vi "Read Line detector configuration.vi"(8 "error in (no error)":errorcluster, 11 "Line Detector in":refnum<class "Resonance Detector.lvclass">) -> (0 "error out":errorcluster, 2 "Configuration":T1={"Peak width guess"=0.0, "Background removal"=enum."NONE", "Smoothing"=enum."NONE", "Smooth window"=100.0, "Relative threshold"=0.0, "Finder algorithm"=enum."Basic", "Bgd window"=100.0, "Spectrum recorder module name"="Spectrum Recorder", "Fit window"=100.0, "Initial fit guess"=enum."Peak finder", "Follow\npeaks"=FALSE, "Re-sample"=nan} {"Re-sample" format="%#_6pHz"; "Fit window" format="%#_6pHz"; "Bgd window" format="%#_6pHz"; "Smooth window" format="%#_6pHz"; "Peak width guess" format="%#_6pHz"}, 3 "Line Detector out":refnum<class "Resonance Detector.lvclass">)   [LabVIEW 2016, in "Resonance Detector.lvclass"]
uses:
  Resonance Detector.lvclass
  C:/github/LabActor/Template Module/Template Module.lvclass
  Resonance Detector Configuration.ctl
  Template Module/Template Module.lvclass/Template Module.ctl
  Template Module/Read Configuration.vi
panel:
  # "Peak finder config"
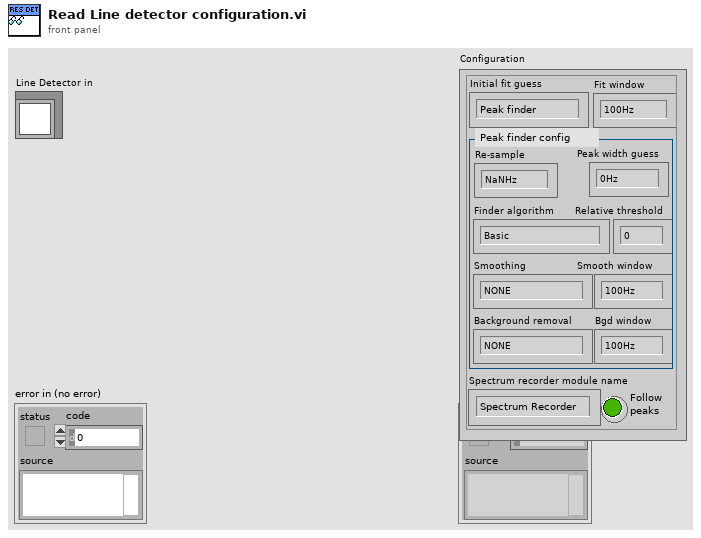
[diagram p1: front panel]
types:
  T1 = typedef "Resonance Detector Configuration.ctl" = cluster{"Peak width guess":dbl, "Background removal":enum16{"NONE", "High-pass", "Detrend"}, "Smoothing":enum16{"NONE", "Low-pass", "Denoise"}, "Smooth window":dbl, "Relative threshold":dbl, "Finder algorithm":enum16{"Basic", "Wavelet", "Wavelet+detrend"}, "Bgd window":dbl, "Spectrum recorder module name":string, "Fit window":dbl, "Initial fit guess":enum16{"Peak finder", "Last fit"}, "Follow\npeaks":bool, "Re-sample":dbl}
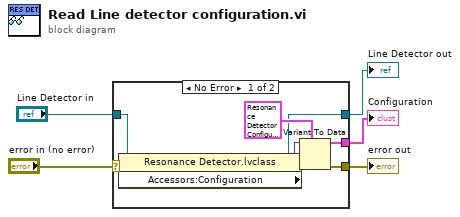
[diagram p0: block diagram]
diagram:
  n1 = case shown="No Error" "error in (no error)" {
    selector: "error in (no error)" -> [w13 w14]
    tunnel: [w12 w14] -> w4
    tunnel: [w7 w15] -> w2
    tunnel: "Line Detector in" -> [w8 w15]
    tunnel: [w10 _] -> w1
    frame No Error {
      n2 = property class="Resonance Detector.lvclass"(reference=w8, error in=w13) -> (reference out=w7:refnum<class "Resonance Detector.lvclass">, error out=w9:errorcluster, "Accessors:Configuration"=w6:variant)
      n3 = Variant To Data(error in=w9, type=T1 {"Peak width guess"=0.0, "Background removal"=enum."NONE", "Smoothing"=enum."NONE", "Smooth window"=100.0, "Relative threshold"=0.0, "Finder algorithm"=enum."Basic", "Bgd window"=100.0, "Spectrum recorder module name"="Spectrum Recorder", "Fit window"=100.0, "Initial fit guess"=enum."Peak finder", "Follow\npeaks"=FALSE, "Re-sample"=nan} ("Configuration"), Variant=w6) -> (data=w10:T1, error out=w12:errorcluster)
    }
    frame Error {
    }
  }
  "error out" <- w4
  "Line Detector out" <- w2
  "Configuration" <- w1
